vi "Set Probe Angle and Offset.vi"(9 "Probe Select":i32, 10 "Probe.Offset":dbl, 11 "Probe.Angle":dbl) -> ()   [LabVIEW 2015, in "Tool Cfg.lvlib"]
uses:
  Tool Cfg.lvlib
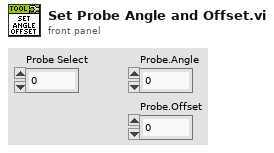
[diagram p1: front panel]
types:
  T1 = typedef "Tool Cfg.lvlib/_ProbeConfigParams Cluster--typedef.ctl" = cluster{"Name":string, "Laser Init Pwr":u16, "Laser Gain":u8, "Integ Count":u16, "Meas. Range":sgl, "Angle":sgl, "Probe Offset":sgl, "Sensor Block":T2}
  T2 = typedef "Tool Cfg.lvlib/_Sensor Block Cluster--typedef.ctl" = cluster{"nSensors":u16, "SensorCfgParams Array":T3[]}
  T3 = typedef "Tool Cfg.lvlib/_SensorConfigParams Cluster--typedef.ctl" = cluster{"Total Pixels":u16, "Positive  Peaks":bool, "CalibrCoefArray":dbl[], "Start Idx":u16, "End Idx":u16}
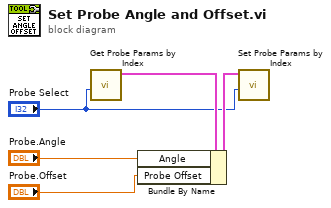
[diagram p0: block diagram]
diagram:
  n1 = call "Get Probe Params by Index.vi"("Probe Select"="Probe Select") -> ("Probe Cfg Params"=w5:T1)  [unwired: 10 in]
  n2 = Bundle By Name(cluster=w5, "Angle"="Probe.Angle", "Probe Offset"="Probe.Offset") -> (w2:T1)
  n3 = call "Set Probe Params by Index.vi"("Index"="Probe Select", "Probe Cfg Params"=w2) -> ()  [unwired: 10 in]
